vi "CloseAllWatchdogs.vi"(8 "error in (no error)":errorcluster, 11 "Pound in":refnum<class "Pound.lvclass">) -> (0 "error out":errorcluster, 3 "Pound out":refnum<class "Pound.lvclass">)   [LabVIEW 2017, in "Pound.lvclass"]
doc: "Close all of the currently active watchdogs. Does not close the pack."
uses:
  <vilib>/NI/Software Watchdog/Pound/Pound.lvclass
  <vilib>/NI/Software Watchdog/Watchdog/Watchdog.lvclass
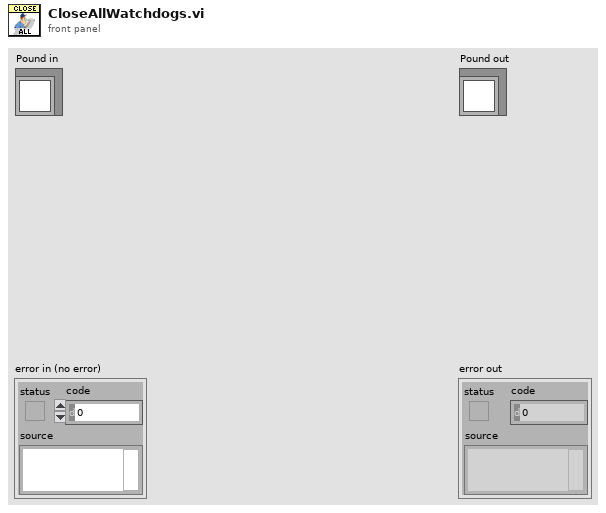
[diagram p1: front panel]
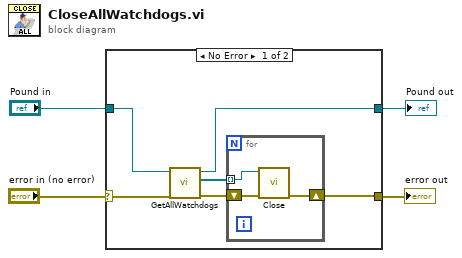
[diagram p0: block diagram]
diagram:
  n1 = case shown="No Error" "error in (no error)" {
    selector: "error in (no error)" -> [w5 w15]
    tunnel: [w6 w15] -> w3
    tunnel: [w7 w14] -> w1
    tunnel: "Pound in" -> [w8 w14]
    frame No Error {
      n2 = call <vilib>:"GetAllWatchdogs.vi"("error in (no error)"=w5, "Pound in"=w8) -> ("error out"=w10:errorcluster, "All Watchdogs"=w9:refnum<data-value>[], "Pound out"=w7:refnum<class "Pound.lvclass">)  [unwired: 7 in]
      n3 = for {
        tunnel: w9 -> [w13] mode=indexing
        shift-right: [w11] -> w6
        shift-left: w10 -> [w12]
        n4 = call <vilib>:"Close.vi"("error in (no error)"=w12, "Watchdog"=w13) -> ("error out"=w11:errorcluster)  [unwired: 9 in]
      }
    }
    frame Error {
    }
  }
  "error out" <- w3
  "Pound out" <- w1
